vi "Victory Message.vi"(11 "MyTeam in":refnum<class "MyTeam.lvclass">) -> (2 "Victory Message":string)   [LabVIEW 2020, in "SquareTeam.lvlib" / "MyTeam.lvclass"]
uses:
  MyTeam.lvclass
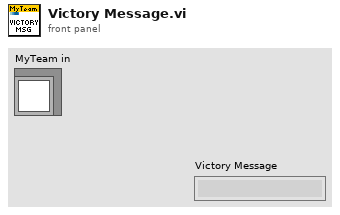
[diagram p1: front panel]
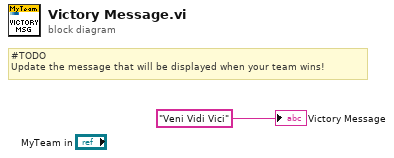
[diagram p0: block diagram]
diagram:
  # "#TODO\nUpdate the message that will be displayed when your team wins!"
  "Victory Message" <- "Veni Vidi Vici" ("Victory Message")
